vi "Disconnect SV.vi"(8 "error in (no error)":errorcluster, 9 "Event Registration Refnum":refnum<event-registration>, 10 "Shared Variables":refnum<k21>[](array[refnum]), 11 "User Event in":refnum<user-event>) -> (0 "error out":errorcluster)   [LabVIEW 2016, in "SMD-7615.lvlib"]
doc: "This VI disconnects Shared Variables and unregisters the specific User Event."
uses:
  SMD-7615.lvlib
  <vilib>/lvdsc/NI_DSC.lvlib
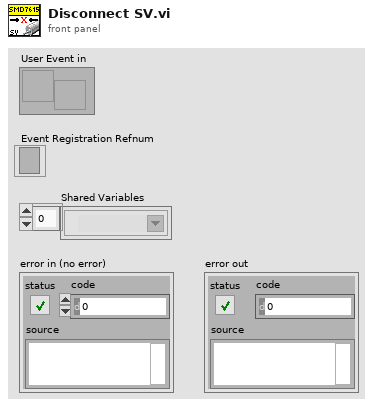
[diagram p1: front panel]
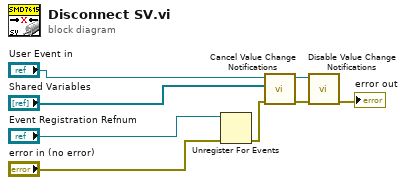
[diagram p0: block diagram]
diagram:
  n1 = Unregister For Events(event registration refnum="Event Registration Refnum", error in="error in (no error)") -> (error out=w3:errorcluster)
  n2 = call <vilib>:"Cancel Value Change Notifications.vi"("error in (no error)"=w3, "shared variables"="Shared Variables", "notification refnum"="User Event in") -> ("error out"=w1:errorcluster, "shared variable value change notification"=w2:refnum<user-event>)  [unwired: 7 out]
  n3 = call <vilib>:"Disable Value Change Notifications.vi"("error in (no error)"=w1, "notification refnum"=w2) -> ("error out"=→"error out":errorcluster)  [unwired: 9 out]
